vi "Launch Debugger.vi"(8 "error in (no error)":errorcluster, 10 "Parent In":refnum<class "Module.lvclass">, 11 "Debug Launcher in":refnum<class "Debug Launcher.lvclass">) -> (0 "error out":errorcluster, 2 "Parent":refnum<class "Module.lvclass">)   [LabVIEW 2020, in "Volatus.lvlib" / "Debug Launcher.lvclass"]
uses:
  Debug Launcher.lvclass
  Module/Module.lvclass
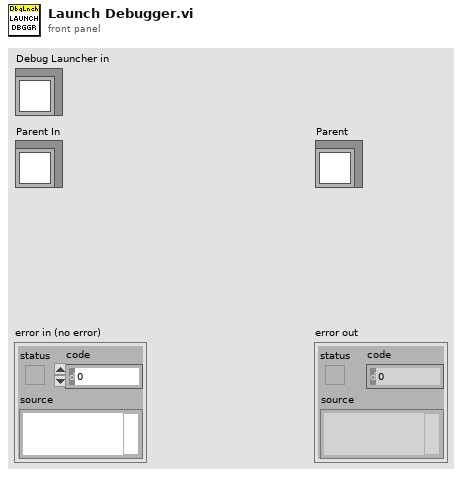
[diagram p1: front panel]
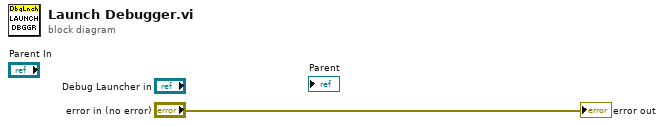
[diagram p0: block diagram]
diagram:
  "error out" <- "error in (no error)"
